vi "Write DebuggingTerminal.vi"(8 "error in (no error)":errorcluster, 10 "DebuggingTerminal":refnum<class "DebuggingTerminal.lvclass">, 11 "Session in":refnum<class "Session.lvclass">) -> (0 "error out":errorcluster, 3 "Session out":refnum<class "Session.lvclass">)   [LabVIEW 2013, in "MQTT Base.lvlib" / "Session.lvclass"]
uses:
  Session.lvclass
  DebuggingTerminal/DebuggingTerminal.lvclass
  Session.lvclass/Session.ctl
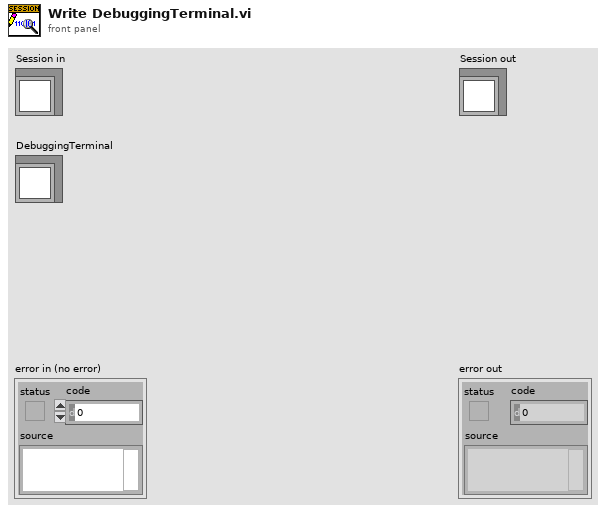
[diagram p1: front panel]
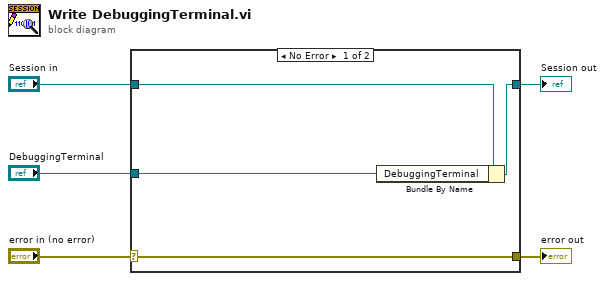
[diagram p0: block diagram]
diagram:
  n1 = case shown="No Error" "error in (no error)" {
    selector: "error in (no error)" -> [w9 w10]
    tunnel: [w9 w10] -> w4
    tunnel: [w7 w11] -> w2
    tunnel: "Session in" -> [w8 w11]
    tunnel: "DebuggingTerminal" -> [w6 _]
    frame No Error {
      n2 = Bundle By Name(cluster=w8, "DebuggingTerminal"=w6) -> (w7:refnum<class "Session.lvclass">)
    }
    frame Error {
    }
  }
  "error out" <- w4
  "Session out" <- w2
